vi "Calibration Control Loop 2016.vi"   [LabVIEW 2015]
uses:
  <vilib>/Rock Robotics/Network Tables/SD Read Boolean.vi
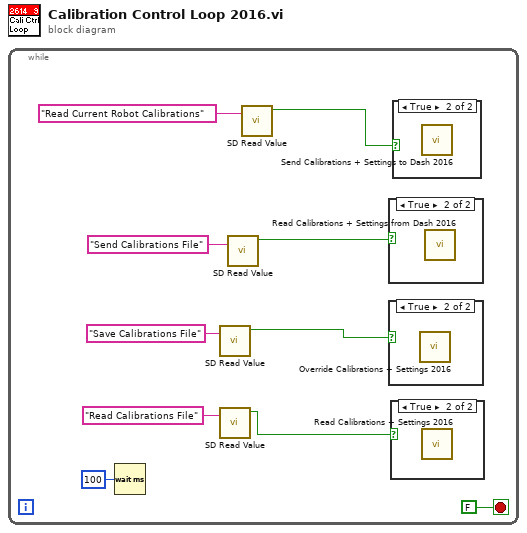
[diagram p0: block diagram]
diagram:
  n1 = while {
    stop <- FALSE stop-if-true
    n2 = Wait (ms)(milliseconds to wait=u32 100) -> ()  [unwired: 1 out]
    n3 = call-poly <vilib>:"SD Read Value.vi"("Name"="Save Calibrations File") -> ("Boolean"=w5:bool)  [unwired: 8 in, 2 out]
    n4 = call-poly <vilib>:"SD Read Value.vi"("Name"="Read Calibrations File") -> ("Boolean"=w3:bool)  [unwired: 8 in, 2 out]
    n5 = call-poly <vilib>:"SD Read Value.vi"("Name"="Send Calibrations File") -> ("Boolean"=w7:bool)  [unwired: 8 in, 2 out]
    n6 = call-poly <vilib>:"SD Read Value.vi"("Name"="Read Current Robot Calibrations") -> ("Boolean"=w9:bool)  [unwired: 8 in, 2 out]
    n7 = case shown="True" w7 {
      frame False {
      }
      frame True {
        n8 = call "Read Calibrations + Settings from Dash 2016.vi"() -> ()  [unwired: 12 in]
      }
    }
    n9 = case shown="True" w5 {
      frame False {
      }
      frame True {
        n10 = call "Override Calibrations + Settings 2016.vi"() -> ()  [unwired: 12 in]
      }
    }
    n11 = case shown="True" w3 {
      frame False {
      }
      frame True {
        n12 = call "Read Calibrations + Settings 2016.vi"() -> ()  [unwired: 12 in]
      }
    }
    n13 = case shown="True" w9 {
      frame False {
      }
      frame True {
        n14 = call "Send Calibrations + Settings to Dash 2016.vi"() -> ()  [unwired: 12 in]
      }
    }
  }
